vi "Diagnostics.vi"() -> ()   [LabVIEW 2019]
doc: "Use this template to build a producer/consumer design pattern. Use this template when you need to execute a process, such as data analysis, when a data source, such as a triggered acquisition, produces data at an uneven rate and you need to execute the process when the data becomes available."
uses:
  <vilib>/DAQmx/create/channels.llb/DAQmx Create Channel (AI-Voltage-Basic).vi
  <vilib>/DAQmx/configure/timing.llb/DAQmx Timing (Sample Clock).vi
  <vilib>/DAQmx/read.llb/DAQmx Read (Analog 1D Wfm NChan NSamp).vi
  <vilib>/express/express analysis/Spectral/Block/exnSpectralBlock spectral measurements RMS poly.vi
  <vilib>/express/express analysis/Spectral/XNode/ExpressSpectralMeasurementsBlockNode.xnode
  <vilib>/measure/NI_MAPro.lvlib
  <vilib>/express/express analysis/Spectral/Block/exnSpectralBlock spectral measurements RMS WFM.vi
  <vilib>/measure/madcrms.llb/Basic Averaged DC-RMS for 1 Chan.vi
panel:
  in  "Spectrum axis":i32
  out "Signal waveforms":waveform(dbl)[](graph)
  out "Signal spectrum":cluster{"f0":dbl, "df":dbl, "magnitude":dbl[]}(graph)
  out "Elapsed Time (s)":dbl
  in  "Endpoint":string
  in  "Recording time":dbl=15.0 caption="Time Target (s)"
  in  "Sample rate":dbl=10000.0 format="%#_13g"
  in  "Samples per channel":i32=10000
  in  "stop":bool
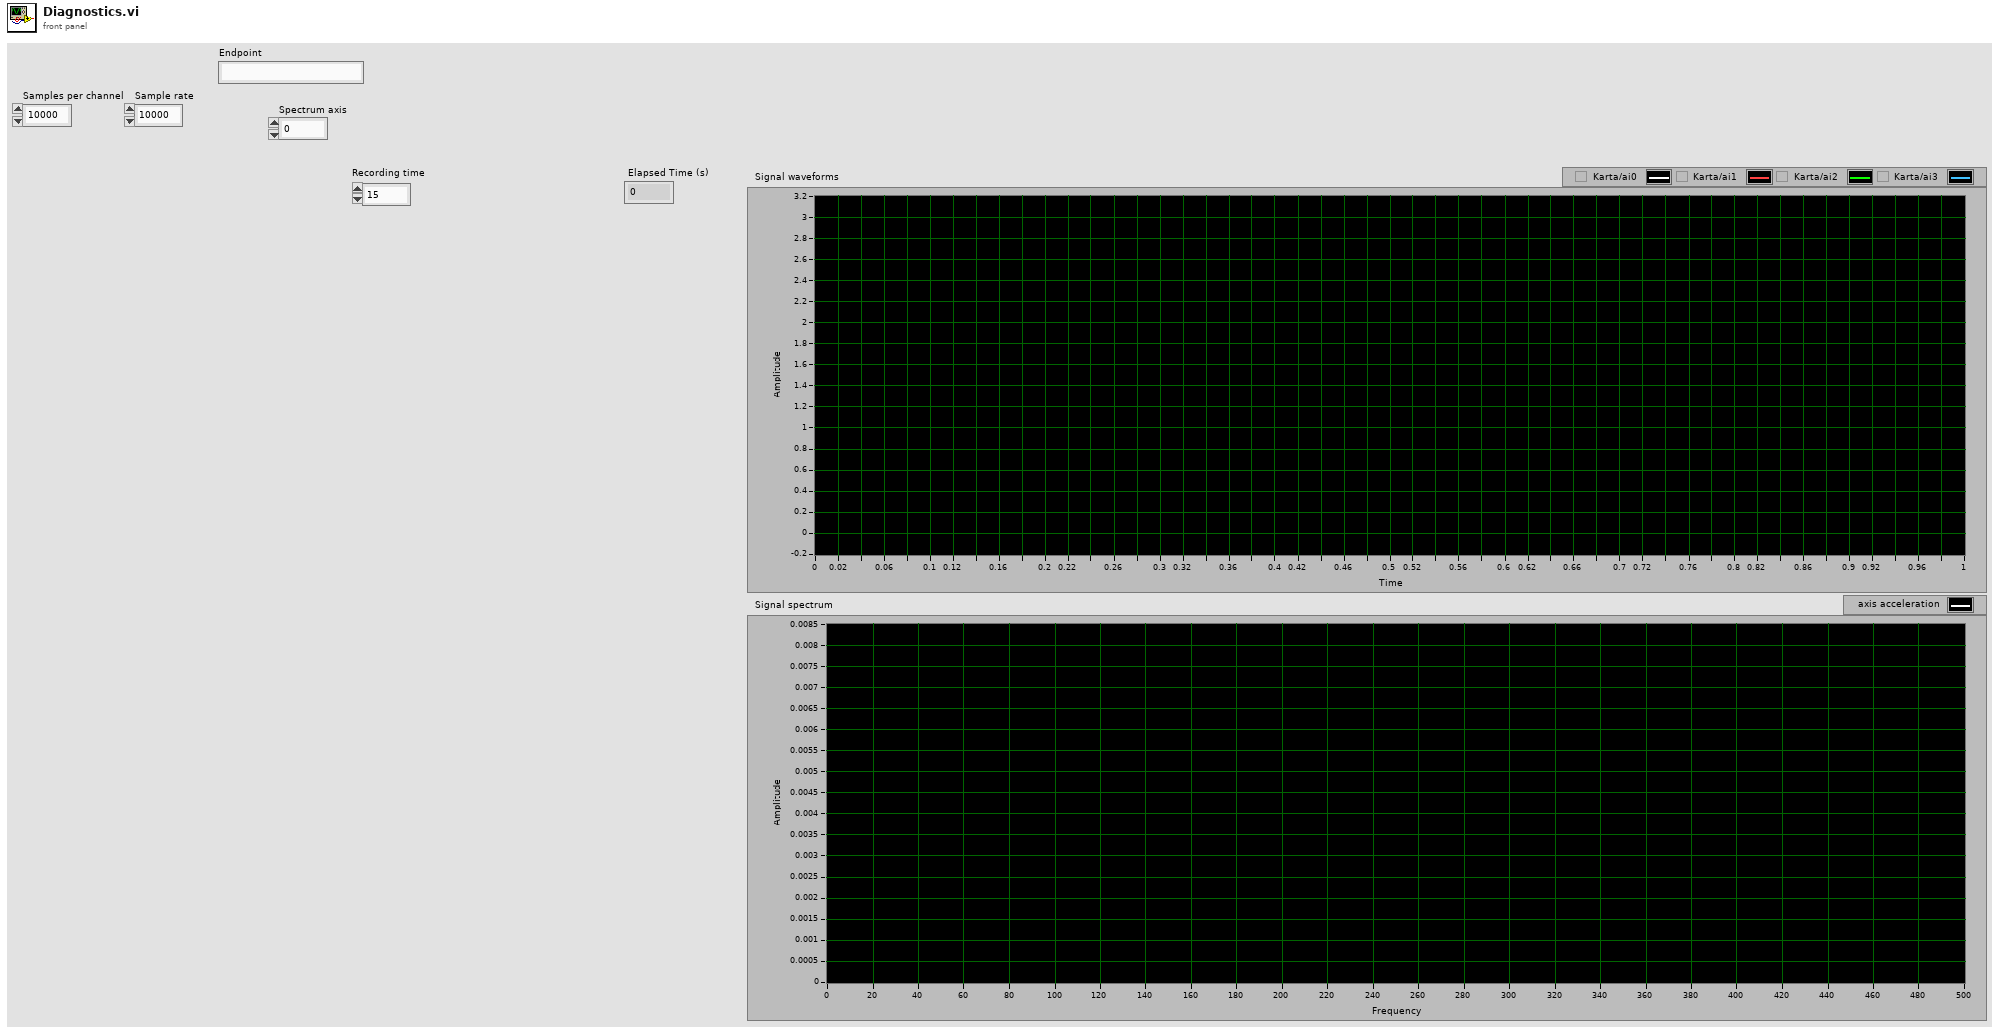
[diagram p1: front panel]
types:
  T1 = cluster{"averaging mode":u16, "weighting mode":u16, "number of averages":u32}
  T2 = cluster{"dB On (F)":bool, "unwrap phase (F)":bool, "convert to degree (F)":bool}
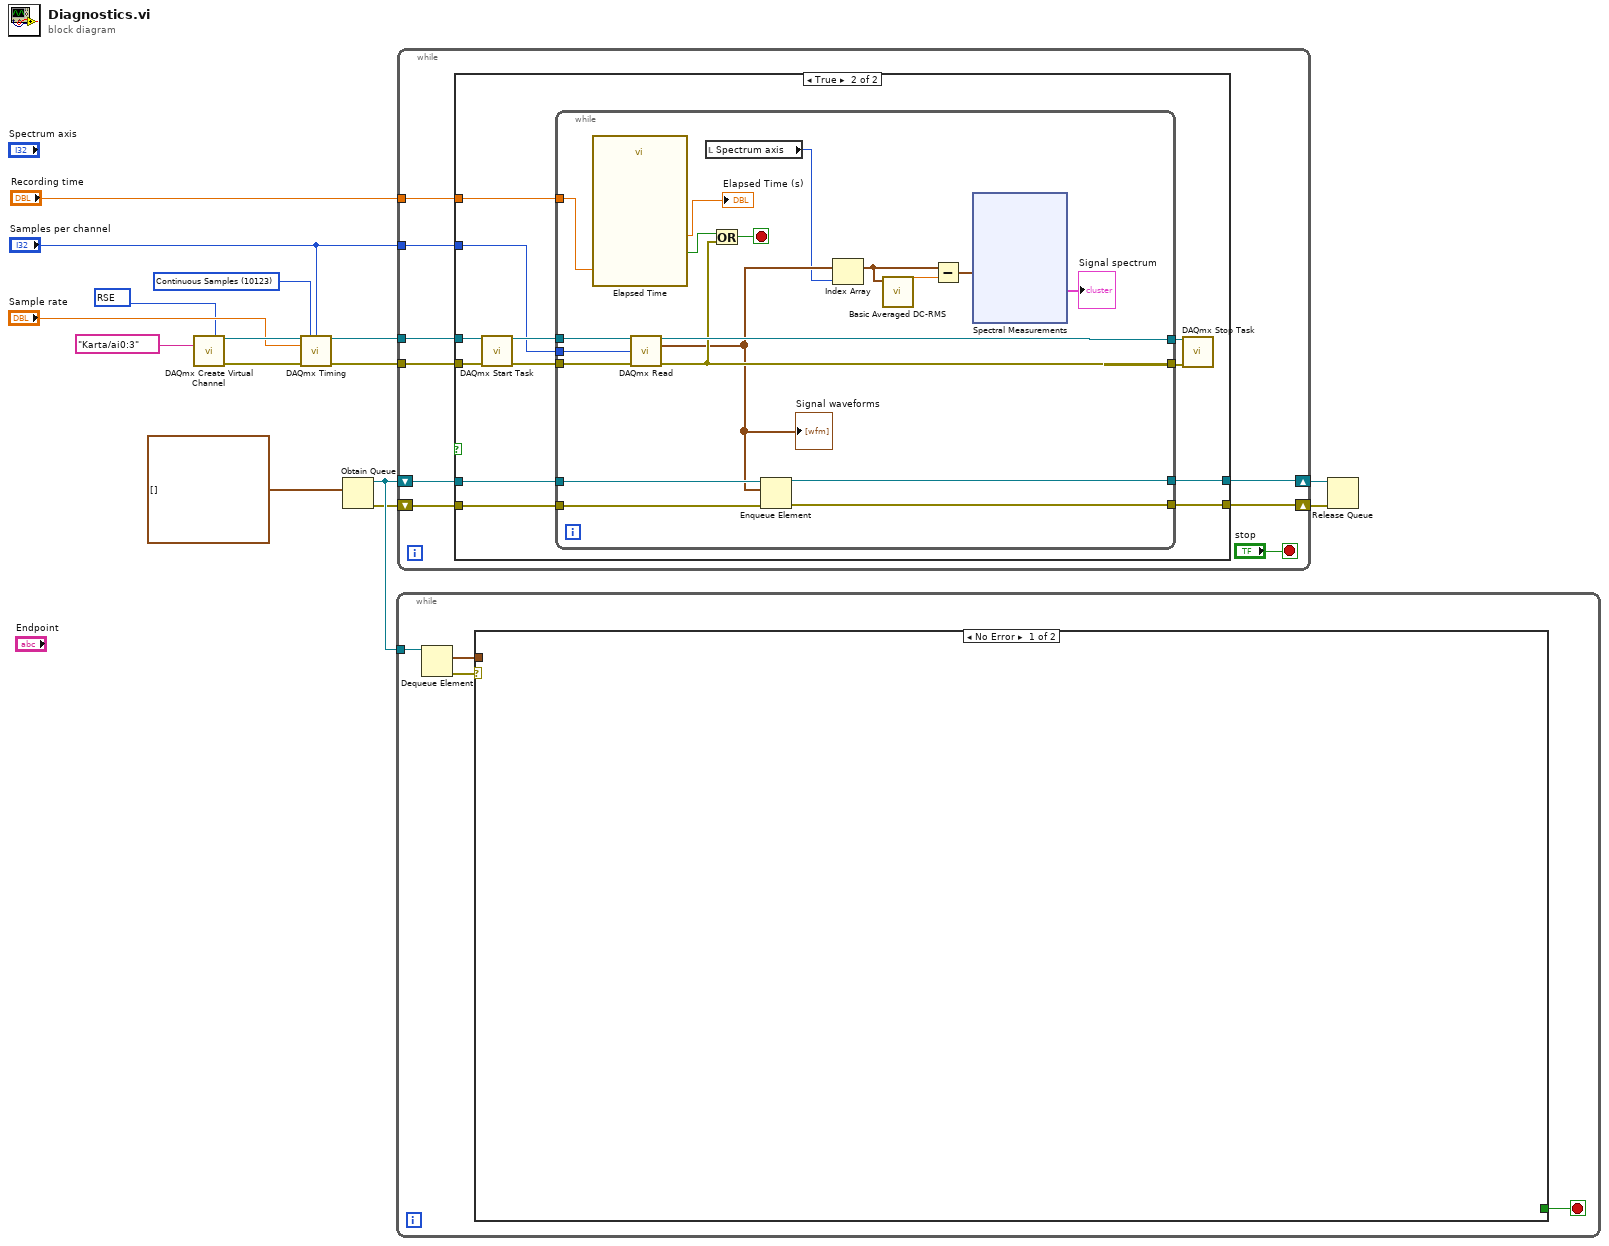
[diagram p0: block diagram]
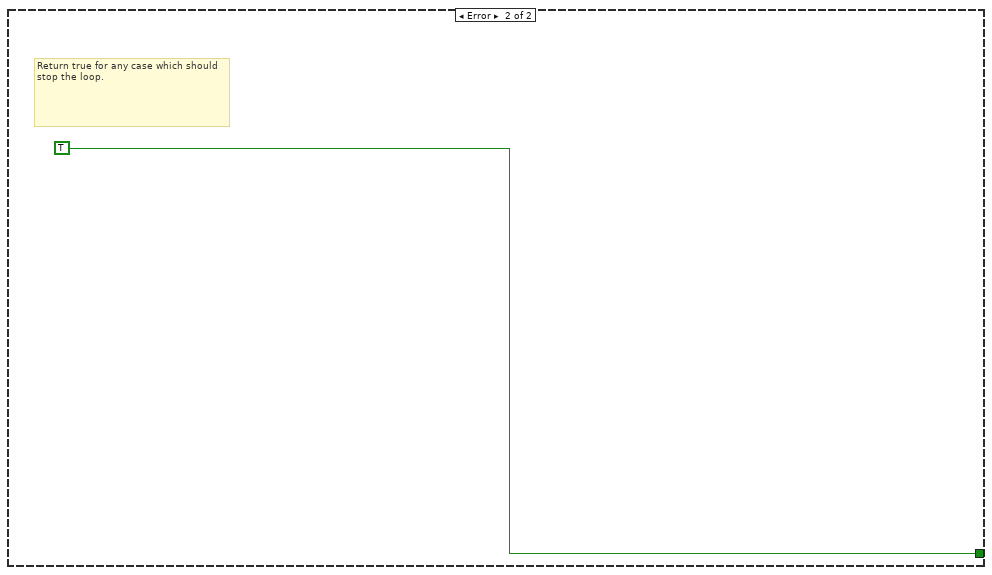
[diagram p2: hidden frame]
diagram:
  w6 = 10083 items=["Default"=-1, "RSE"=10083, "NRSE"=10078, "Differential"=10106, "Pseudodifferential"=12529] ("input terminal configuration")
  w8 = 10123 items=["Finite Samples"=10178, "Continuous Samples"=10123, "Hardware Timed Single Point"=12522] ("sample mode")
  n1 = call-poly <vilib>:"DAQmx Create Virtual Channel.vi"("input terminal configuration"=w6, "physical channels"=tag "Karta/ai0:3") -> ("task out"=w9:refnum<k21>, "error out"=w10:errorcluster)  [unwired: 12 in]
  n2 = call-poly <vilib>:"DAQmx Timing.vi"("task/channels in"=w9, "sample mode"=w8, "samples per channel"="Samples per channel", "rate"="Sample rate", "error in"=w10) -> ("task out"=w4:refnum<k21>, "error out"=w3:errorcluster)  [unwired: 9 in]
  n3 = Obtain Queue(element data type=waveform(dbl)[] [] ("data")) -> (queue out=w15:refnum<queue>, error out=w14:errorcluster)  [unwired: 4 in, 1 out]
  n4 = while {
    tunnel: w15 -> [w19]
    stop <- w16 stop-if-true
    n5 = Dequeue Element(queue=w19) -> (element=w17:waveform(dbl)[], error out=w18:errorcluster)  [unwired: 2 in, 2 out]
    n6 = case shown="No Error" w18 {
      tunnel: w17 -> [_ _]
      tunnel: [_ TRUE] -> w16
      frame No Error {
      }
      frame Error {
        # "Return true for any case which should stop the loop."
      }
    }
  }
  n7 = while {
    shift-right: [w25] -> w12
    shift-left: w14 -> [w26]
    shift-right: [w27] -> w13
    shift-left: w15 -> [w28]
    tunnel: w4 -> [w24]
    tunnel: w3 -> [w23]
    tunnel: "Samples per channel" -> [w22]
    tunnel: "Recording time" -> [w21]
    stop <- "stop" stop-if-true
    n8 = case shown="True" {
      selector: _ -> [_ _]
      tunnel: w28 -> [w31 w35]
      tunnel: [w31 w32] -> w27
      tunnel: w26 -> [w30 w34]
      tunnel: [w30 w33] -> w25
      tunnel: w24 -> [_ w43]
      tunnel: w23 -> [_ w42]
      tunnel: w22 -> [_ w39]
      tunnel: w21 -> [_ w38]
      frame False {
      }
      frame True {
        n9 = call <vilib>:"DAQmx Start Task.vi"("task/channels in"=w43, "error in"=w42) -> ("task out"=w41:refnum<k21>, "error out"=w40:errorcluster)  [unwired: 12 in]
        n10 = while {
          tunnel: w41 -> [w62]
          tunnel: w40 -> [w61]
          tunnel: w39 -> [w60]
          tunnel: w38 -> [w59]
          tunnel: [w55] -> w37
          tunnel: [w54] -> w36
          tunnel: w35 -> [w53]
          tunnel: w34 -> [w52]
          tunnel: [w51] -> w33
          tunnel: [w50] -> w32
          stop <- w56 stop-if-true
          n11 = call "Elapsed Time"("Time Target (s)"=w59) -> ("Elapsed Time (s)"=→"Elapsed Time (s)":dbl, "Time has Elapsed"=w57:bool)  [unwired: 11 in, 6 out]
          n12 = call-poly <vilib>:"DAQmx Read.vi"("task/channels in"=w62, "number of samples per channel"=w60, "error in"=w61) -> ("task out"=w55:refnum<k21>, "data"=w45:waveform(dbl)[], "error out"=w54:errorcluster)  [unwired: 10 in]
          "Signal waveforms" <- w45
          n13 = local read "Spectrum axis"() -> (w44:i32)
          n14 = Or(x=w57, y=w54) -> (x .or. y?=w56:bool)
          n15 = Enqueue Element(queue=w53, element=w45, error in (no error)=w52) -> (queue out=w50:refnum<queue>, error out=w51:errorcluster)  [unwired: 1 in, 1 out]
          n16 = Index Array(array=w45, index=w44) -> (element=w48:waveform(dbl))
          n17 = call-poly <vilib>:"Basic Averaged DC-RMS.vi"("signal in"=w48) -> ("DC value"=w46:dbl)  [unwired: 7 in, 3 out]
          n18 = Subtract(x=w48, y=w46) -> (x-y=w47:waveform(dbl))
          n19 = xnode "Spectral Measurements"("Signals"=w47) -> ("FFT - (RMS)"=→"Signal spectrum":cluster{"f0":dbl, "df":dbl, "magnitude":dbl[]})  [unwired: 1 in, 2 out]
        }
        n20 = call <vilib>:"DAQmx Stop Task.vi"("task/channels in"=w37, "error in"=w36) -> ()  [unwired: 12 in, 2 out]
      }
    }
  }
  n21 = Release Queue(queue=w13, error in (no error)=w12) -> ()  [unwired: 1 in, 3 out]
